vi "init.vi"(8 "error in":errorcluster, 10 "TBM module configuration in":refnum<class "TBM module configuration.lvclass">, 11 "Benchmark PID runtime in":refnum<class "Benchmark PID runtime.lvclass">) -> (0 "error out":errorcluster, 1 "data allocations":T1, 2 "execution settings":T4, 3 "Benchmark PID runtime out":refnum<class "Benchmark PID runtime.lvclass">)   [LabVIEW 2018, in "Benchmark PID runtime.lvclass"]
doc: "Provides an interface for initializing a module at runtime. While this interface performs no operations, a child should provide an override which may open any necessary references or sessions, allocate necessary memory, and perform any final configuration validataion before providing the full configuration <b>execution data</b> to the calling process."
uses:
  Benchmark PID runtime.lvclass
  <vilib>/NI/Tag Bus Module Framework/channel/TBM channel.lvclass
  <vilib>/NI/Tag Bus Module Framework/runtime/TBM module execution interface.lvclass
  configuration/Benchmark PID configuration.lvclass
  <vilib>/NI/Tag Bus/dictionary/data dictionary.lvclass
  Mappings.ctl
  C:/Program Files (x86)/National Instruments/LabVIEW 2018/vi.lib/NI/Tag Bus/tag/tag descriptor.lvclass
  <vilib>/NI/Tag Bus Module Framework/module configuration/TBM module configuration.lvclass
  <vilib>/NI/Tag Bus Module Framework/runtime/execution settings.ctl
  <vilib>/NI/Tag Bus Module Framework/channel/data tables.ctl
  <vilib>/NI/Tag Bus/dictionary table pair.ctl
  <vilib>/NI/Tag Bus/tag bus.lvlib
  <vilib>/NI/Tag Bus/table/data table.ctl
  <vilib>/NI/Tag Bus/table/data table.lvlib
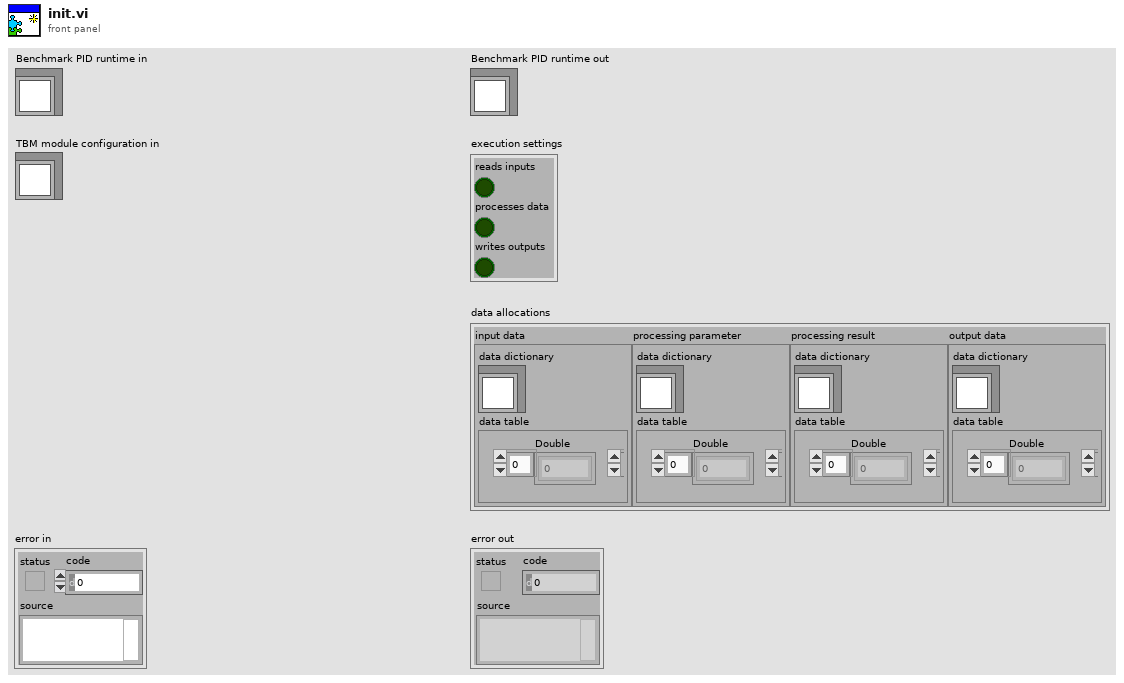
[diagram p1: front panel]
types:
  T1 = typedef "TBM channel.lvclass/data tables.ctl" = cluster{"input data":T2, "processing parameter":T2, "processing result":T2, "output data":T2}
  T2 = typedef "tag bus.lvlib/dictionary table pair.ctl" = cluster{"data dictionary":refnum<class "data dictionary.lvclass">, "data table":T3}
  T3 = typedef "tag bus.lvlib/data table.lvlib/data table.ctl" = cluster{"Double":dbl[], "Single":sgl[], "I64":i64[], "I32":i32[], "I16":i16[], "I8":i8[], "U64":u64[], "U32":u32[], "U16":u16[], "U8":u8[], "Boolean":bool[], "String":string[], "Array of Double":cluster{"DBL Array":dbl[]}[], "Array of Single":cluster{"SGL Array":sgl[]}[], "Array of I64":cluster{"I64 Array":i64[]}[], "Array of I32":cluster{"I32 Array":i32[]}[], "Array of I16":cluster{"I16 Array":i16[]}[], "Array of I8":cluster{"I8 Array":i8[]}[], "Array of U64":cluster{"U64 Array":u64[]}[], "Array of U32":cluster{"U32 Array":u32[]}[], "Array of U16":cluster{"U16 Array":u16[]}[], "Array of U8":cluster{"U8 Array":u8[]}[], "Array of Boolean":cluster{"Boolean Array":bool[]}[], "Array of String":cluster{"String Array":string[]}[]}
  T4 = typedef "TBM module execution interface.lvclass/execution settings.ctl" = cluster{"reads inputs":bool, "processes data":bool, "writes outputs":bool}
  T5 = cluster{"proportional gain (Kc)":dbl, "integral time (Ti, min)":dbl, "derivative time (Td, min)":dbl}
  T6 = typedef "Mappings.ctl" = cluster{"Setpoint Index":i32, "Variable Index":i32, "Output Index":i32}
  T7 = typedef "Benchmark PID configuration.lvclass/Line.ctl" = cluster{"PID Name":string, "Setpoint":refnum<class "TBM channel.lvclass">, "Variable":refnum<class "TBM channel.lvclass">, "Output":refnum<class "TBM channel.lvclass">}
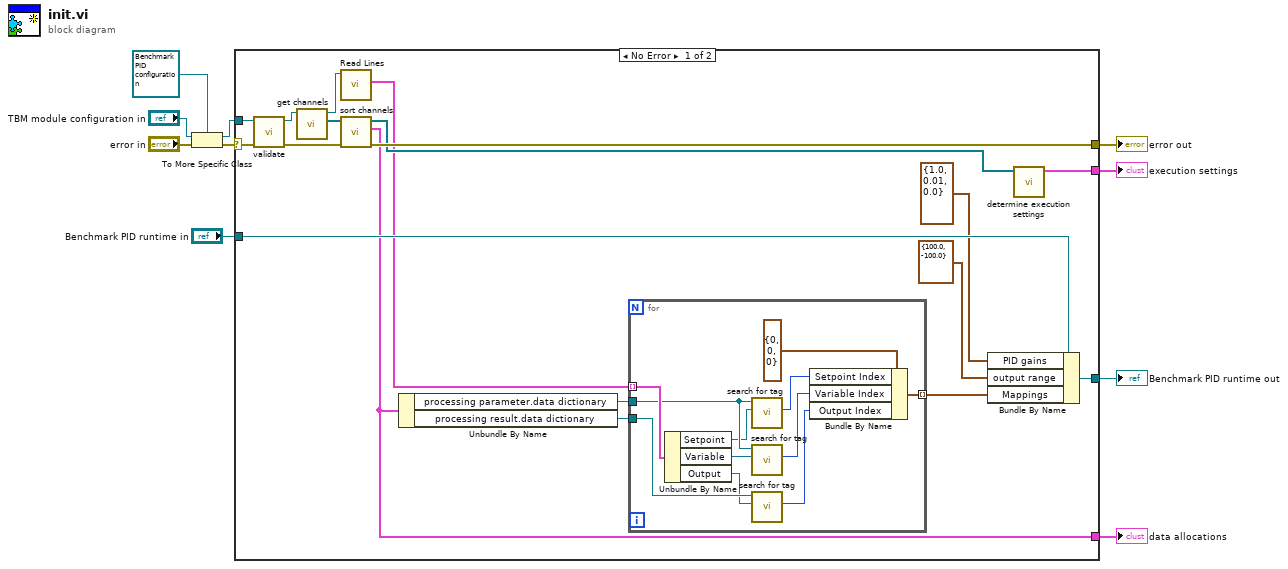
[diagram p0: block diagram]
diagram:
  n1 = To More Specific Class(target class=refnum<class "Benchmark PID configuration.lvclass"> refnum ("Synchronous module configuration"), reference="TBM module configuration in", error in="error in") -> (specific class reference=w9:refnum<class "Benchmark PID configuration.lvclass">, error out=w10:errorcluster)
  n2 = case shown="No Error" w10 {
    selector: w10 -> [w23 w40]
    tunnel: w9 -> [w22 _]
    tunnel: "Benchmark PID runtime in" -> [w28 w41]
    tunnel: [w19 w41] -> w4
    tunnel: [w27 w40] -> w3
    tunnel: [w14 _] -> w1
    tunnel: [w26 _] -> w2
    frame No Error {
      n3 = call-dynamic "validate.vi"("error in"=w23, "Benchmark PID configuration in"=w22) -> ("error out"=w24:errorcluster, "Benchmark PID configuration out"=w21:refnum<class "Benchmark PID configuration.lvclass">)  [unwired: 8 in]
      n4 = call-dynamic "get channels.vi"("Benchmark PID configuration in"=w21) -> ("channels"=w20:refnum<class "TBM channel.lvclass">[], "Benchmark PID configuration out"=w16:refnum<class "Benchmark PID configuration.lvclass">)  [unwired: 9 in]
      n5 = call "Read Lines.vi"("Benchmark PID configuration in"=w16) -> ("Lines"=w15:T7[])  [unwired: 8 in, 2 out]
      n6 = call <vilib>:"sort channels.vi"("error in"=w24, "channels in"=w20) -> ("error out"=w27:errorcluster, "data allocations"=w14:T1, "channels out"=w25:refnum<class "TBM channel.lvclass">[])  [unwired: 7 in]
      n7 = Unbundle By Name(w14) -> ("processing parameter.data dictionary"=w13:refnum<class "data dictionary.lvclass">, "processing result.data dictionary"=w12:refnum<class "data dictionary.lvclass">)
      n8 = for {
        tunnel: w15 -> [w39] mode=indexing
        tunnel: w13 -> [w38]
        tunnel: w12 -> [w37]
        tunnel: [w29] -> w11 mode=indexing
        n9 = Unbundle By Name(w39) -> ("Setpoint"=w36:refnum<class "TBM channel.lvclass">, "Variable"=w35:refnum<class "TBM channel.lvclass">, "Output"=w34:refnum<class "TBM channel.lvclass">)
        n10 = call <vilib>:"search for tag.vi"("system tag"=w36, "data dictionary in"=w38) -> ("index"=w32:i32)  [unwired: 7 in, 2 out]
        n11 = call <vilib>:"search for tag.vi"("system tag"=w35, "data dictionary in"=w38) -> ("index"=w31:i32)  [unwired: 7 in, 2 out]
        n12 = call <vilib>:"search for tag.vi"("system tag"=w34, "data dictionary in"=w37) -> ("index"=w30:i32)  [unwired: 7 in, 2 out]
        n13 = Bundle By Name(cluster=T6 {"Setpoint Index"=0, "Variable Index"=0, "Output Index"=0} ("output cluster"), "Setpoint Index"=w32, "Variable Index"=w31, "Output Index"=w30) -> (w29:T6)
      }
      n14 = Bundle By Name(cluster=w28, "PID gains"=T5 {"proportional gain (Kc)"=1.0, "integral time (Ti, min)"=0.01, "derivative time (Td, min)"=0.0}, "output range"=cluster{"output high":dbl, "output low":dbl} {"output high"=100.0, "output low"=-100.0}, "Mappings"=w11) -> (w19:refnum<class "Benchmark PID runtime.lvclass">)
      n15 = call <vilib>:"determine execution settings.vi"("channels"=w25) -> ("execution settings"=w26:T4)  [unwired: 10 in]
    }
    frame Error {
    }
  }
  "error out" <- w3
  "Benchmark PID runtime out" <- w4
  "execution settings" <- w2
  "data allocations" <- w1
